vi "test_acquire_image (single).vi"(11 "PicamModel":T1=715 items=["---PIXIS 100 SERIES---"=1000, "PixisSeries"=0, "Pixis100BR"=5, "---PI-MAX4 SERIES---"=1001, "Pimax4Series"=700, "PiMax41024EM"=715]) -> (0 "error out":errorcluster, 2 "first pixel":u16)   [LabVIEW 2019, in "Picam.lvclass"]
uses:
  Picam.lvclass
  picam32_LabView_SDK/PICam_lib/types/PicamModel.ctl
panel:
  in  "error in (no error)":errorcluster
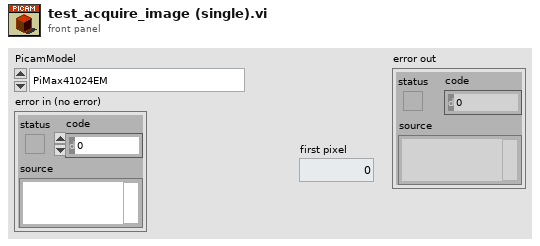
[diagram p1: front panel]
types:
  T1 = typedef "PicamModel.ctl" = u32
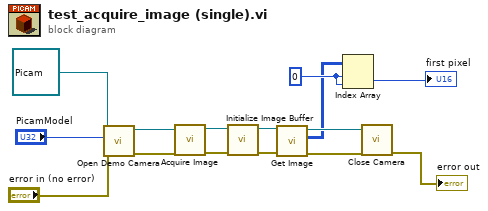
[diagram p0: block diagram]
diagram:
  w3 = 0 ("index (row)")
  n1 = call-dynamic "Open Demo Camera.vi"("error in (no error)"="error in (no error)", "PicamModel"="PicamModel", "Picam in"=refnum<class "Picam.lvclass"> refnum) -> ("error out"=w12:errorcluster, "Picam out"=w11:refnum<class "Picam.lvclass">)  [unwired: 7 in]
  n2 = call-dynamic "Acquire Image.vi"("error in (no error)"=w12, "Picam in"=w11) -> ("error out"=w10:errorcluster, "Picam out"=w8:refnum<class "Picam.lvclass">)  [unwired: 8 in]
  n3 = call-dynamic "Initialize Image Buffer.vi"("error in (no error)"=w10, "Picam in"=w8) -> ("error out"=w7:errorcluster, "Picam out"=w6:refnum<class "Picam.lvclass">)  [unwired: 8 in]
  n4 = call-dynamic "Get Image.vi"("error in (no error)"=w7, "Picam in"=w6) -> ("error out"=w5:errorcluster, "Image"=w2:u16[][], "Picam out"=w4:refnum<class "Picam.lvclass">)  [unwired: 7 in]
  n5 = Index Array(array=w2, index (row)=w3, index (col)=w3) -> (element=→"first pixel":u16)
  n6 = call-dynamic "Close Camera.vi"("error in (no error)"=w5, "Picam in"=w4) -> ("error out"=→"error out":errorcluster)  [unwired: 8 in, 1 out]
